vi "GetClassProperties.vi"(0 "reference in":refnum<class "ClassWriterNative.lvclass">, 1 "LvClassItem":refnum<vi>, 2 "TreeControl":refnum<vi>, 5 "error in (no error)":errorcluster) -> (14 "reference out":refnum<class "ClassWriterNative.lvclass">, 19 "error out":errorcluster)   [LabVIEW 2020, in "ClassWriterNative.lvclass"]
uses:
  <resource>/Framework/Providers/Open_GDS/ClassProviders/Provider_LvNativeClass/ClassWriterNative_class/ClassWriterNative.lvclass
panel:
  out "ObjectClasses":string[](array[string])
  out "ObjectAttributes":string[][](array[string])
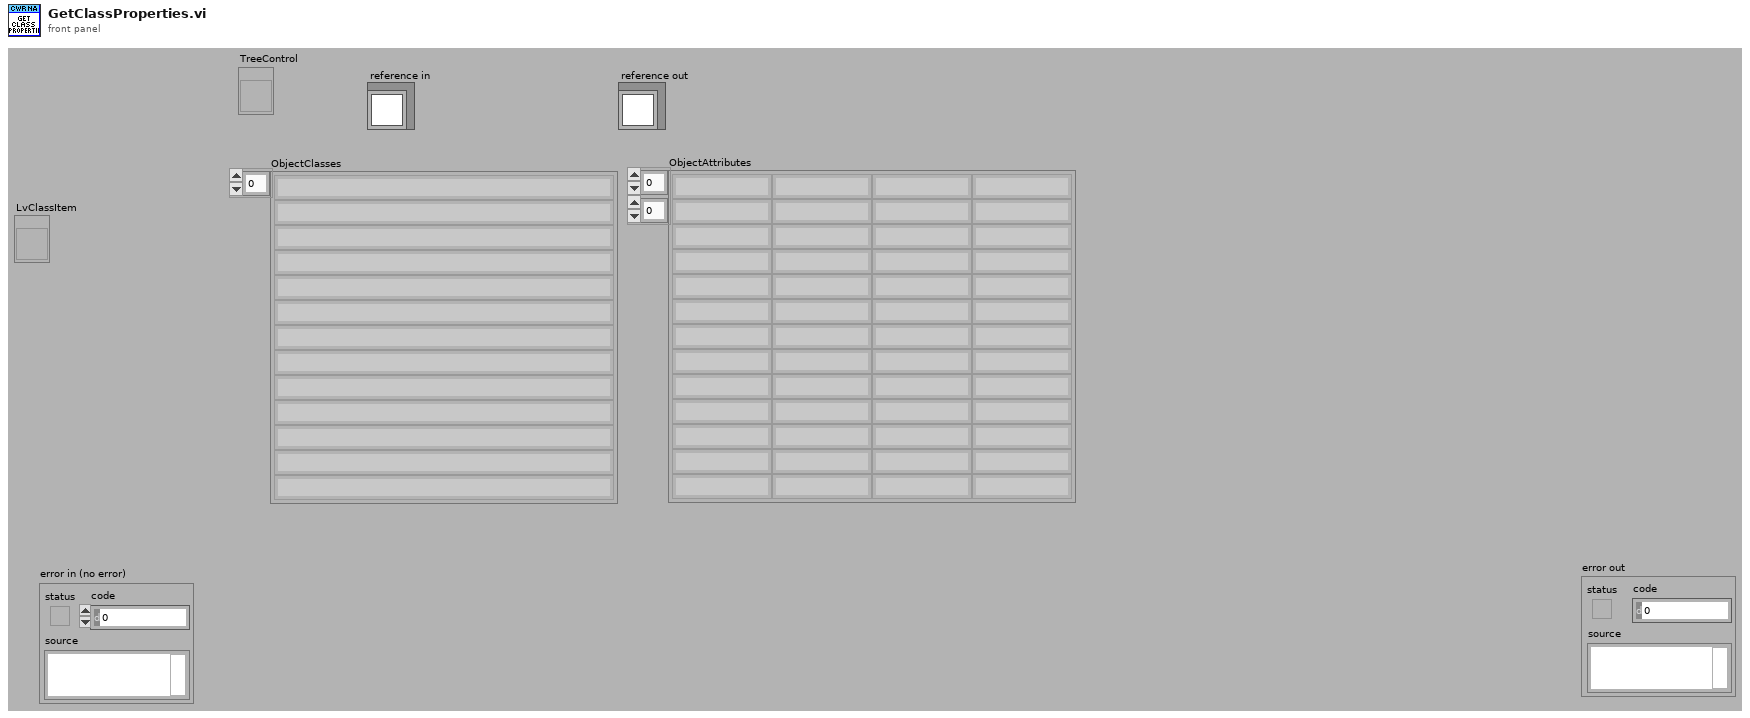
[diagram p1: front panel]
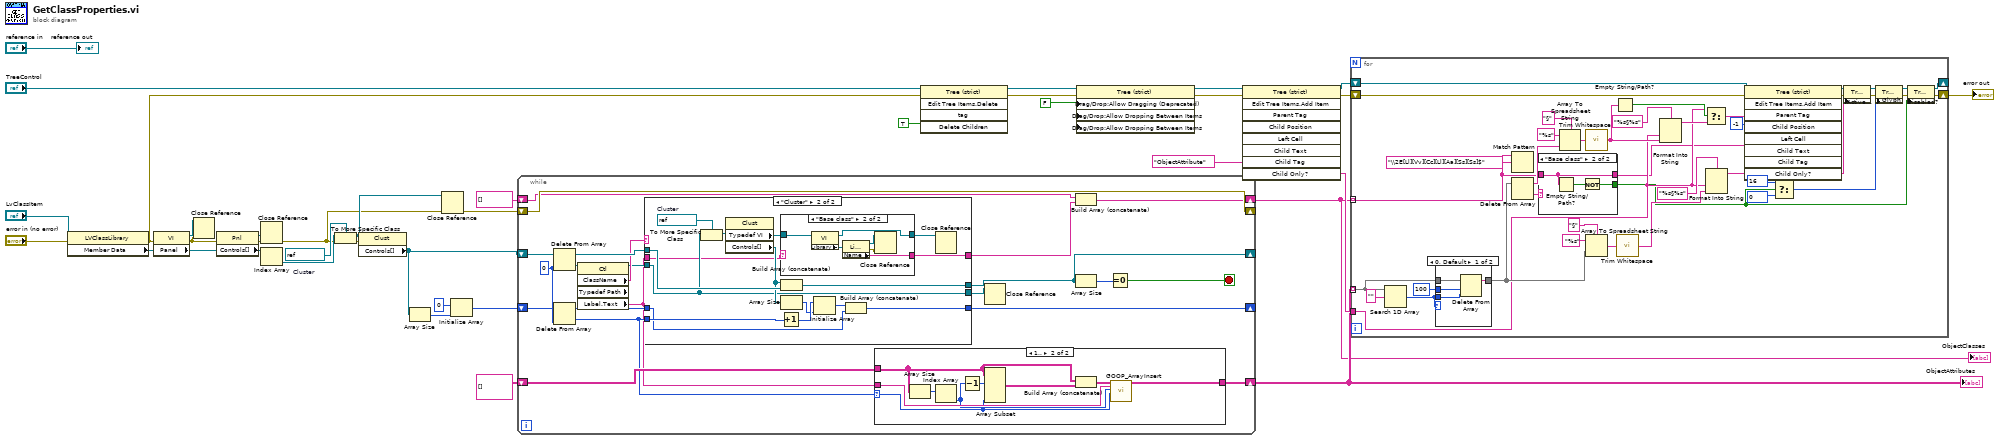
[diagram p0: block diagram]
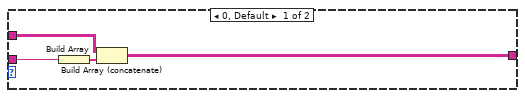
[diagram p2: hidden frame]
diagram:
  w12 = refnum<vi> refnum  # Cluster
  w30 = FALSE ("Drag/Drop:Allow Dragging (Deprecated)")
  w28 = "ObjectAttribute" ("Left Cell String(Main name)")
  n1 = property class="LVClassLibrary"(reference="LvClassItem", error in="error in (no error)") -> (error out=w19:errorcluster, "Member Data"=w20:refnum<vi>)  [unwired: 1 out]
  n2 = property class="VI"(reference=w20, error in=w19) -> (reference out=w7:refnum<vi>, error out=w8:errorcluster, "Panel"=w18:refnum<vi>)
  n3 = Close Reference(reference=w7, error in (no error)=w8) -> ()  [unwired: 1 out]
  n4 = property class="Pnl"(reference=w18, error in=w8) -> (reference out=w2:refnum<vi>, error out=w4:errorcluster, "Controls[]"=w13:refnum<vi>[])
  n5 = Close Reference(reference=w2, error in (no error)=w4) -> (error out=w3:errorcluster)
  n6 = Index Array(array=w13) -> (element=w11:refnum<vi>)  [unwired: 1 in]
  n7 = To More Specific Class(target class=w12, reference=w11, error in=w3) -> (specific class reference=w6:refnum<vi>, error out=w10:errorcluster)
  n8 = property class="Clust"(reference=w6, error in=w10) -> ("Controls[]"=w9:refnum<vi>[])  [unwired: 2 out]
  n9 = Array Size(array=w9) -> (size(s)=w16:i32)
  n10 = Close Reference(reference=w6, error in (no error)=w3) -> (error out=w5:errorcluster)
  n11 = Initialize Array(0 ("index"), w16) -> (w14:i32[])
  n12 = while {
    shift-right: [w55] -> _
    shift-left: w9 -> [w57]
    shift-right: [w42] -> _
    shift-left: w5 -> [w42]
    shift-right: [w50] -> w25
    shift-left: string[][] [] -> [w51]
    shift-right: [w44] -> _
    shift-left: w14 -> [w46]
    shift-right: [w39] -> w24
    shift-left: string[] [] -> [w40]
    stop <- w53 stop-if-true
    w47 = 0 ("index")
    n13 = Delete From Array(array=w57, index=w47) -> (deleted portion=w52:refnum<vi>, array with subset deleted=w56:refnum<vi>[])  [unwired: 1 in]
    n14 = Delete From Array(array=w46, index=w47) -> (deleted portion=w43:i32, array with subset deleted=w45:i32[])  [unwired: 1 in]
    n15 = property class="Ctl" props=["ClassName", "Typedef Path", "Label", "Text"](reference=w52) -> (reference out=w48:refnum<vi>, "ClassName"=w49:string, "Label.Text"=w37:string)  [unwired: 1 in, 2 out]
    n16 = case shown="\"Cluster\"" w49 {
      tunnel: [w73 w87] -> w55
      tunnel: w56 -> [w73 w86]
      tunnel: w48 -> [w71 w78]
      tunnel: w45 -> [w72 w80]
      tunnel: [w72 w81] -> w44
      tunnel: w43 -> [_ w84]
      tunnel: [w71 w78] -> w41
      tunnel: [_ w76] -> w38
      tunnel: w37 -> [_ w74]
      frame Default {
      }
      frame "Cluster" {
        w89 = refnum<vi> refnum  # Cluster
        n17 = To More Specific Class(target class=w89, reference=w78) -> (specific class reference=w88:refnum<vi>)  [unwired: 1 in, 1 out]
        n18 = property class="Clust"(reference=w88) -> ("Typedef VI"=w77:refnum<vi>, "Controls[]"=w85:refnum<vi>[])  [unwired: 1 in, 2 out]
        n19 = Increment(x=w84) -> (x+1=w83:i32)
        n20 = case shown="\"Base class\"" w74 {
          tunnel: w77 -> [w90 w96]
          tunnel: [_ w94] -> w76
          tunnel: [w90 w91] -> w75
          frame "False", Default {
          }
          frame "Base class" {
            n21 = property class="VI"(reference=w96) -> (reference out=w91:refnum<vi>, "Library"=w95:refnum<vi>)  [unwired: 1 in, 1 out]
            n22 = property class="Library"(reference=w95) -> (reference out=w93:refnum<vi>, error out=w92:errorcluster, "Name"=w94:string)  [unwired: 1 in]
            n23 = Close Reference(reference=w93, error in (no error)=w92) -> ()  [unwired: 1 out]
          }
        }
        n24 = Build Array (concatenate)(w85, w86) -> (w87:refnum<vi>[])
        n25 = Array Size(array=w85) -> (size(s)=w82:i32)
        n26 = Initialize Array(w83, w82) -> (w79:i32[])
        n27 = Build Array (concatenate)(w79, w80) -> (w81:i32[])
        n28 = Close Reference(reference=w75) -> ()  [unwired: 1 in, 1 out]
      }
    }
    n29 = case shown="1.." w43 {
      selector: w43 -> [_ w62]
      tunnel: w51 -> [w61 w66]
      tunnel: [w60 w69] -> w50
      tunnel: w37 -> [w59 w68]
      frame 0, Default {
        n30 = Build Array(w59) -> (w58:string[])
        n31 = Build Array (concatenate)(w61, w58) -> (w60:string[][])
      }
      frame 1.. {
        n32 = Array Size(array=w66) -> (size(s)=w70:i32[])
        n33 = Index Array(array=w70) -> (element=w64:i32)  [unwired: 1 in]
        n34 = Decrement(x=w64) -> (x-1=w63:i32)
        n35 = Array Subset(array=w66, index (row)=w63, length (col)=w62) -> (w65:string[][])  [unwired: 2 in]
        n36 = Build Array (concatenate)(w66, w65) -> (w67:string[][])
        n37 = call <resource>:"GOOP_ArrayInsert.vi"("ArrayIn"=w67, "Text"=w68, "Row"=w64, "Column"=w62) -> ("ArrayOut"=w69:string[][])  [unwired: 15 in]
      }
    }
    n38 = Close Reference(reference=w41) -> ()  [unwired: 1 in, 1 out]
    n39 = Build Array (concatenate)(w40, w38) -> (w39:string[])
    n40 = Array Size(array=w55) -> (size(s)=w54:i32)
    n41 = Equal To 0?(x=w54) -> (x = 0?=w53:bool)
  }
  "ObjectAttributes" <- w25
  "ObjectClasses" <- w24
  n42 = invoke on="Invoke Node" class="Tree (strict)" method="Edit Tree Items.Delete"(reference="TreeControl", error in=w19, "Delete Children"=TRUE) -> (reference out=w34:refnum<vi>, error out=w33:errorcluster)  [unwired: 2 in, 3 out]
  n43 = property class="Tree (strict)"(reference=w34, error in=w33, "Drag/Drop:Allow Dragging (Deprecated)"=w30, "Drag/Drop:Allow Dropping Between Items"=w30, "Drag/Drop:Allow Dropping Between Items"=w30) -> (reference out=w32:refnum<vi>, error out=w31:errorcluster)
  n44 = invoke on="Invoke Node" class="Tree (strict)" method="Edit Tree Items.Add Item"(reference=w32, error in=w31, "Left Cell"=w28, "Child Tag"=w28) -> (reference out=w27:refnum<vi>, error out=w26:errorcluster)  [unwired: 5 in, 7 out]
  n45 = for {
    shift-right: [w99] -> w21
    shift-left: w26 -> [w116]
    shift-right: [w98] -> _
    shift-left: w27 -> [w115]
    tunnel: w25 -> [w135] mode=indexing
    tunnel: w28 -> [w118]
    tunnel: w24 -> [w105] mode=indexing
    n46 = Search 1D Array(1D array=w135, element="") -> (index of element=w124:i32)  [unwired: 1 in]
    n47 = case shown="0, Default" w124 {
      tunnel: w124 -> [w144 _]
      tunnel: w135 -> [w143 w145]
      tunnel: 100 ("length") -> [w142 _]
      tunnel: [w141 w145] -> w125
      frame 0, Default {
        n48 = Delete From Array(array=w143, length=w142, index=w144) -> (array with subset deleted=w141:string[])  [unwired: 1 out]
      }
      frame -1 {
      }
    }
    n49 = Match Pattern(string=w105, regular expression="\\2E[Ll][Vv][Cc][Ll][Aa][Ss][Ss]$") -> ()  [unwired: 1 in, 4 out]
    n50 = Delete From Array(array=w125) -> (deleted portion=w113:string, array with subset deleted=w133:string[])  [unwired: 2 in]
    n51 = case shown="\"Base class\"" w113 {
      selector: w113 -> [w137 _]
      tunnel: [w137 w138] -> w112
      tunnel: w105 -> [_ w138]
      tunnel: [_ w139] -> w97
      frame Default {
      }
      frame "Base class" {
        n52 = Empty String/Path?(string/path=w138) -> (empty?=w140:bool)
        n53 = Not(x=w140) -> (.not. x?=w139:bool)
      }
    }
    n54 = Array To Spreadsheet String(delimiter (Tab)="§", array=w133, 3:"%s" ("format string")) -> (spreadsheet string=w130:string)
    n55 = call <vilib>:"Trim Whitespace.vi"("string"=w130) -> ("trimmed string"=w122:string)  [unwired: 1 in]
    n56 = Array To Spreadsheet String(delimiter (Tab)="§", array=w125, 3:"%s" ("format string")) -> (spreadsheet string=w128:string)
    n57 = Empty String/Path?(string/path=w122) -> (empty?=w129:bool)
    n58 = call <vilib>:"Trim Whitespace.vi"("string"=w128) -> ("trimmed string"=w119:string)  [unwired: 1 in]
    n59 = Format Into String(format string="%s§%s", w118, w122) -> (resulting string=w121:string)  [unwired: 2 in, 1 out]
    n60 = Select(t=w118, s=w129, f=w121) -> (s? t:f=w117:string)
    n61 = Format Into String(format string="%s§%s", w118, w119) -> (resulting string=w106:string)  [unwired: 2 in, 1 out]
    n62 = invoke on="Invoke Node" class="Tree (strict)" method="Edit Tree Items.Add Item"(reference=w115, error in=w116, "Parent Tag"=w117, "Child Position"=-1, "Left Cell"=w112, "Child Tag"=w106) -> (reference out=w108:refnum<vi>, error out=w107:errorcluster)  [unwired: 3 in, 7 out]
    n63 = Select(t=16, s=w97, f=0) -> (s? t:f=w102:i32)
    n64 = property class="Tree (strict)"(reference=w108, error in=w107, "Active Item Tag"=w106) -> (reference out=w110:refnum<vi>, error out=w109:errorcluster)
    n65 = property class="Tree (strict)"(reference=w110, error in=w109, "Glyph"=w102) -> (reference out=w101:refnum<vi>, error out=w100:errorcluster)
    n66 = property class="Tree (strict)"(reference=w101, error in=w100, "Disabled?"=w97) -> (reference out=w98:refnum<vi>, error out=w99:errorcluster)
  }
  "error out" <- w21
  "reference out" <- "reference in"
